vi "Log_Init.vi"(6 "Facilities":string[](array[string])=["Sys", "UI", "Logger", "DAQ", "Data", "DBP", "REST"], 8 "error in (no error)":errorcluster, 9 "Level":T2=enum."error", 10 "Log File":path, 11 "reference in":refnum<class "Log.lvclass"> caption="This control should only be used when\na sub class is inheriting this class") -> (0 "error out":errorcluster, 3 "reference out":refnum<class "Log.lvclass"> caption="This indicator should only be used when\na sub class is inheriting this class")   [LabVIEW 2023, in "Log.lvclass"]
uses:
  Log.lvclass
  Log_Level.ctl
  Log_Facilities.ctl
panel:
  in  "Name":T1="default"
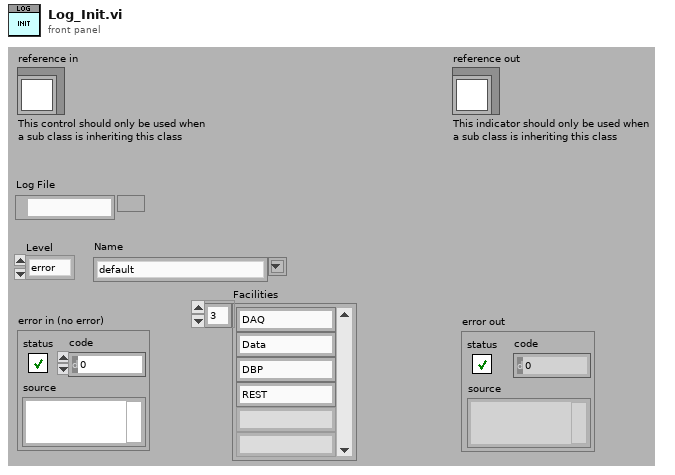
[diagram p1: front panel]
types:
  T1 = typedef "Log.lvclass/Log_Facilities.ctl" = string
  T2 = typedef "Log.lvclass/Log_Level.ctl" = enum16{"none", "info", "trace", "warn", "error", "fatal"}
  T3 = typedef "Log.lvclass/ObjectAttributes.ctl" = cluster{"Level":T2, "Facilities":variant, "Event":refnum<user-event>}
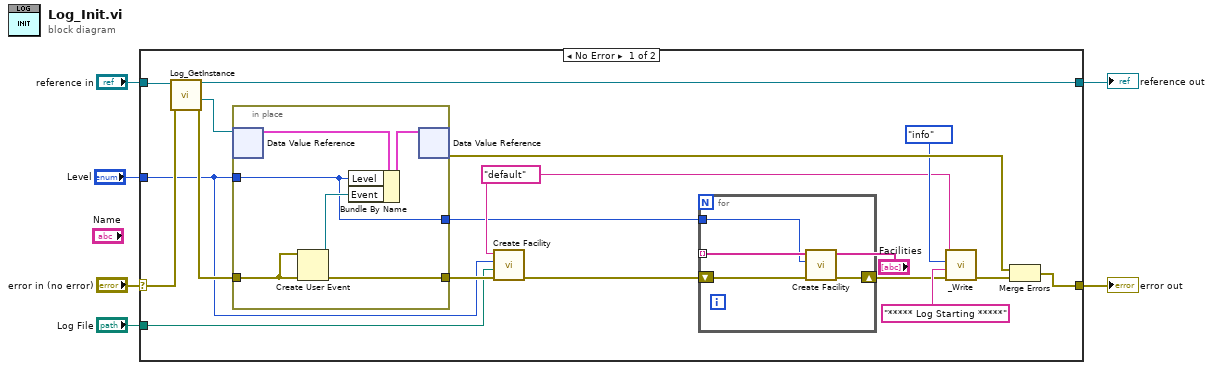
[diagram p0: block diagram]
diagram:
  n1 = case shown="No Error" "error in (no error)" {
    selector: "error in (no error)" -> [w24 w36]
    tunnel: [w19 w36] -> w5
    tunnel: "reference in" -> [w23 w35]
    tunnel: [w21 w35] -> w3
    tunnel: "Log File" -> [w16 _]
    tunnel: "Level" -> [w14 _]
    frame No Error {
      w12 = T1 "default" ("Name")
      n2 = call "Log_GetInstance.vi"("error in (no error)"=w24, "reference in"=w23) -> ("error out"=w20:errorcluster, "DVRRefOut"=w22:refnum<data-value>, "reference out"=w21:refnum<class "Log.lvclass">)  [unwired: 5 in, 2 out]
      n3 = in-place {
        in-place-border: w20 -> [w31]
        in-place-border: [w32] -> w18
        in-place-border: w14 -> [w29]
        in-place-border: [w29] -> w9
        n4 = in-place-dvr #1(w22) -> (w33:T3)  [unwired: 1 out]
        n5 = Create User Event(user event datatype=w31, error in=w31) -> (user event=w30:refnum<user-event>, error out=w32:errorcluster)
        n6 = Bundle By Name(cluster=w33, "Level"=w29, "Event"=w30) -> (w34:T3)
        n7 = in-place-dvr #1(w34) -> (w17:errorcluster)  [unwired: 1 out]
      }
      n8 = call "Create Facility.vi"("error in (no error)"=w18, "Log File (Use default)"=w16, "Level (error)"=w14, "Name"=w12) -> ("error out"=w8:errorcluster)  [unwired: 7 in]
      n9 = for {
        shift-right: [w28] -> w10
        shift-left: w8 -> [w27]
        tunnel: w9 -> [w26]
        tunnel: "Facilities" -> [w25] mode=indexing
        n10 = call "Create Facility.vi"("error in (no error)"=w27, "Level (error)"=w26, "Name"=w25) -> ("error out"=w28:errorcluster)  [unwired: 8 in]
      }
      n11 = call "_Write.vi"("error in (no error)"=w10, "Message"="***** Log Starting *****" ("Name"), "Level"=Log_Level."info", "Name"=w12) -> ("error out"=w15:errorcluster)  [unwired: 7 in]
      n12 = Merge Errors(w17, w15) -> (w19:errorcluster)
    }
    frame Error {
    }
  }
  "error out" <- w5
  "reference out" <- w3
